vi "Table Pick Row Border V2A.vi"(6 "# header rows":i32, 7 "Data Row Back Ground color":T8={"color"=16777225, "at each"=0}, 8 "columnWidth (points)":sgl[](array[numeric]), 9 "Row format with ref [ ]":T7(array[cluster]), 10 "i":i32) -> (0 "columnWidth (points) out":sgl[](array[numeric]), 1 "Row format with ref":T6, 3 "Background Color":u32(colorbox))   [LabVIEW 2019]
doc: "Version 2.0\nDeveloped by Jean-Marc Simard\nCopyright © 2012, Exaprom Inc.\nAll rights reserved.\nLicense: BSD"
uses:
  <userlib>/Exaprom PDF/Controls/Table Controls/Row Back Ground color Datas.ctl
  <userlib>/Exaprom PDF/Controls/Table Controls/Cell Cluster.ctl
  C:/Program Files/National Instruments/LabVIEW 2019/user.lib/Exaprom PDF/DLL/itextsharp.dll
  DLL/itextsharp.dll
  <userlib>/Exaprom PDF/Controls/Text Controls/Unicode/Type and run direction.ctl
  <userlib>/Exaprom PDF/Controls/Table Controls/Cell Alignment 20px.ctl
  <userlib>/Exaprom PDF/Controls/Table Controls/Text vertical arrangement.ctl
  <userlib>/Exaprom PDF/Controls/Font Controls/Font size.ctl
  <userlib>/Exaprom PDF/VIs/Low level/General/Stop if it True.vi
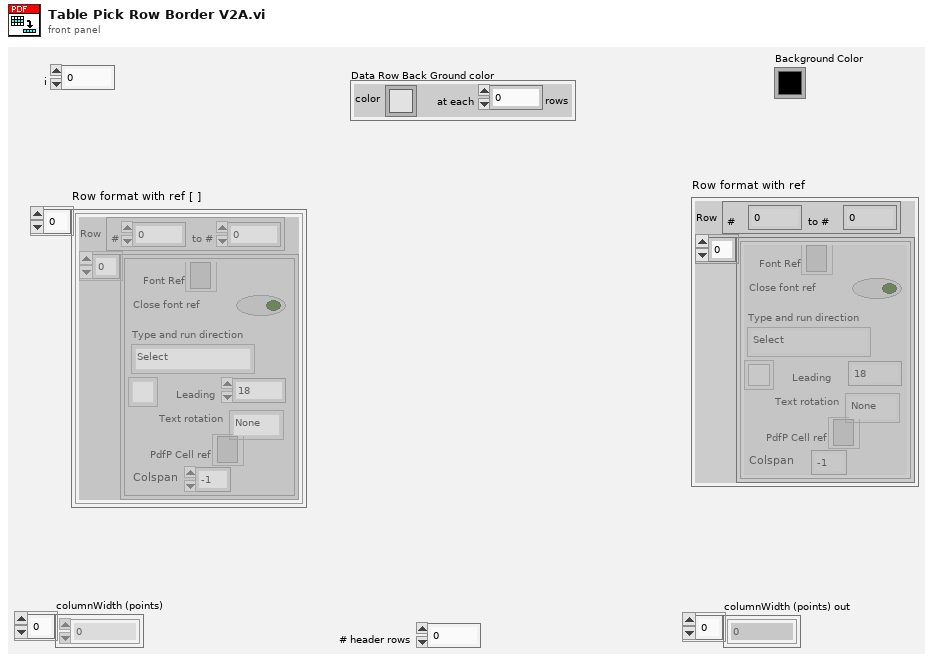
[diagram p1: front panel]
types:
  T1 = typedef "Cell Cluster.ctl" = cluster{"Font Ref":refnum<k24>, "Close font ref":bool, "Type and run direction":T2, "Cell Alignment":T3, "Text rotation":T4, "Leading":T5, "PdfP Cell ref":refnum<k24>, "Colspan":i8}
  T2 = typedef "Type and run direction.ctl" = enum16{"Select", "ASCII", "UTF-16", "UTF-16 (default)", "UTF-16 (LTR)", "UTF-16 (RTL)"}
  T3 = typedef "Cell Alignment 20px.ctl" = u16
  T4 = typedef "Text vertical arrangement.ctl" = enum16{"None", "Clockwise", "Counterclockwise"}
  T5 = typedef "Font size.ctl" = sgl
  T6 = cluster{"Row":cluster{"#":i16, "to #":i16}, "Cell [ ]":T1[]}
  T7 = cluster{"Row":cluster{"#":i16, "to #":i16}, "Cell [ ]":T1[]}[]
  T8 = typedef "Row Back Ground color Datas.ctl" = cluster{"color":u32, "at each":i16}
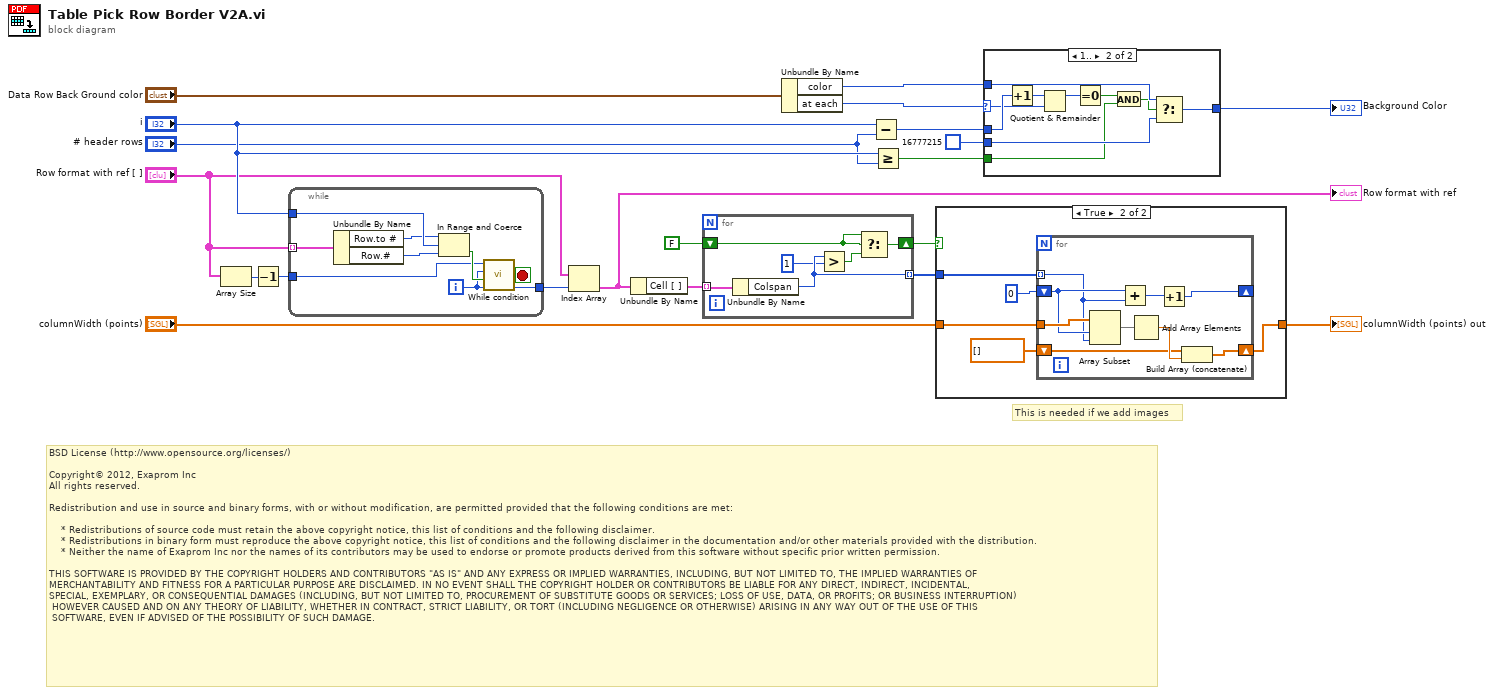
[diagram p0: block diagram]
diagram:
  # "This is needed if we add images"
  # "BSD License (http://www.opensource.org/licenses/)\n\nCopyright© 2012, Exaprom Inc\nAll rights reserved.\n\nRedistribution and use in source and binary forms, with or without modification, are permitted provided that the following conditions are met:\n\n    * Redistributions of source code must retain the above copyright notice, this list of conditions and the following disclaimer.\n    * Redistributions in binary form must reproduce the above copyright notice, this list of conditions and the following disclaimer in the documentation and/or other materials provided with the distribution.\n    * Neither the name of Exaprom Inc nor the names of its contributors may be used to endorse or promote products derived from this software without specific prior written permission.\n\nTHIS SOFTWARE IS PROVIDED BY THE COPYRIGHT HOLDERS AND CONTRIBUTORS \"AS IS\" AND ANY EXPRESS OR IMPLIED WARRANTIES, INCLUDING, BUT NOT LIMITED TO, THE IMPLIED WARRANTIES OF \nMERCHANTABILITY AND FITNESS FOR A PARTICULAR PURPOSE ARE DISCLAIMED. IN NO EVENT SHALL THE COPYRIGHT HOLDER OR CONTRIBUTORS BE LIABLE FOR ANY DIRECT, INDIRECT, INCIDENTAL,\nSPECIAL, EXEMPLARY, OR CONSEQUENTIAL DAMAGES (INCLUDING, BUT NOT LIMITED TO, PROCUREMENT OF SUBSTITUTE GOODS OR SERVICES; LOSS OF USE, DATA, OR PROFITS; OR BUSINESS INTERRUPTION)\n HOWEVER CAUSED AND ON ANY THEORY OF LIABILITY, WHETHER IN CONTRACT, STRICT LIABILITY, OR TORT (INCLUDING NEGLIGENCE OR OTHERWISE) ARISING IN ANY WAY OUT OF THE USE OF THIS\n SOFTWARE, EVEN IF ADVISED OF THE POSSIBILITY OF SUCH DAMAGE."
  n1 = Array Size(array="Row format with ref [ ]") -> (size(s)=w15:i32)
  n2 = Decrement(x=w15) -> (x-1=w14:i32)
  n3 = while {
    tunnel: "Row format with ref [ ]" -> [w28] mode=indexing
    tunnel: "i" -> [w27]
    tunnel: [w22] -> w20
    tunnel: w14 -> [w21]
    i -> [w22]
    stop <- w24 stop-if-true
    n4 = Unbundle By Name(w28) -> ("Row.to #"=w25:i16, "Row.#"=w26:i16)
    n5 = In Range and Coerce(upper limit=w25, x=w27, lower limit=w26) -> (In Range?=w23:bool)  [unwired: 1 out]
    n6 = call-poly <userlib>:"While condition.vi"("Test"=w23, "i"=w22, "N"=w21) -> ("Action"=w24:bool)  [unwired: 5 out]
  }
  n7 = Index Array(array="Row format with ref [ ]", index=w20) -> (element=w9:T6)
  "Row format with ref" <- w9
  n8 = Unbundle By Name(w9) -> ("Cell [ ]"=w8:T1[])
  n9 = for {
    tunnel: w8 -> [w34] mode=indexing
    tunnel: [w30] -> w5 mode=indexing
    shift-right: [w33] -> w6
    shift-left: FALSE -> [w32]
    n10 = Unbundle By Name(w34) -> ("Colspan"=w30:i8)
    n11 = Greater?(x=w30, y=i8 1) -> (0:w31:bool)
    n12 = Select(t=w32, s=w32, f=w31) -> (s? t:f=w33:bool)
  }
  n13 = Unbundle By Name("Data Row Back Ground color") -> ("color"=w18:u32, "at each"=w10:i16)
  n14 = Subtract(x="i", y="# header rows") -> (x-y=w11:i32)
  n15 = Greater Or Equal?(x="i", y="# header rows") -> (x >= y?=w2:bool)
  n16 = case shown="True" w6 {
    tunnel: "columnWidth (points)" -> [w35 w37]
    tunnel: [w35 w36] -> w12
    tunnel: w5 -> [_ w40]
    frame False {
    }
    frame True {
      n17 = for {
        tunnel: w40 -> [w46] mode=indexing
        shift-right: [w45] -> _
        shift-left: i8 0 ("span") -> [w47]
        shift-right: [w41] -> w36
        shift-left: sgl[] [] ("columnWidth (points)") -> [w42]
        tunnel: w37 -> [w49]
        n18 = Array Subset(array=w49, index=w47, length=w46) -> (w44:sgl[])
        n19 = Add(x=w47, y=w46) -> (x+y=w48:i8)
        n20 = Add Array Elements(numeric array=w44) -> (sum=w43:sgl)
        n21 = Increment(x=w48) -> (x+1=w45:i8)
        n22 = Build Array (concatenate)(w42, w43) -> (w41:sgl[])
      }
    }
  }
  "columnWidth (points) out" <- w12
  n23 = case shown="1.." w10 {
    selector: w10 -> [_ w51]
    tunnel: w18 -> [_ w58]
    tunnel: u32 16777215 ("Color") -> [w50 w57]
    tunnel: [w50 w56] -> w16
    tunnel: w2 -> [_ w54]
    tunnel: w11 -> [_ w52]
    frame 0, Default {
    }
    frame 1.. {
      n24 = Increment(x=w52) -> (x+1=w60:i32)
      n25 = Quotient & Remainder(x=w60, y=w51) -> (x-y*floor(x/y)=w59:i32)  [unwired: 1 out]
      n26 = Equal To 0?(x=w59) -> (x = 0?=w55:bool)
      n27 = And(x=w55, y=w54) -> (x .and. y?=w53:bool)
      n28 = Select(t=w58, s=w53, f=w57) -> (s? t:f=w56:u32)
    }
  }
  "Background Color" <- w16
